vi "Example_LabVIEW_Google_Map.vi"() -> ()   [LabVIEW 2020]
panel:
  in  "Your Google Maps API Key":string
  in  "Zoom in":bool
  in  "Zoom Out":bool
  in  "Location List":i32(listbox)
  in  "Home":bool
  in  "Go":bool
  in  "WebBrowser":refnum<k7>(container)
  # "Google-Maps URL API for LabVIEW"
  # "Create by Wiseio"
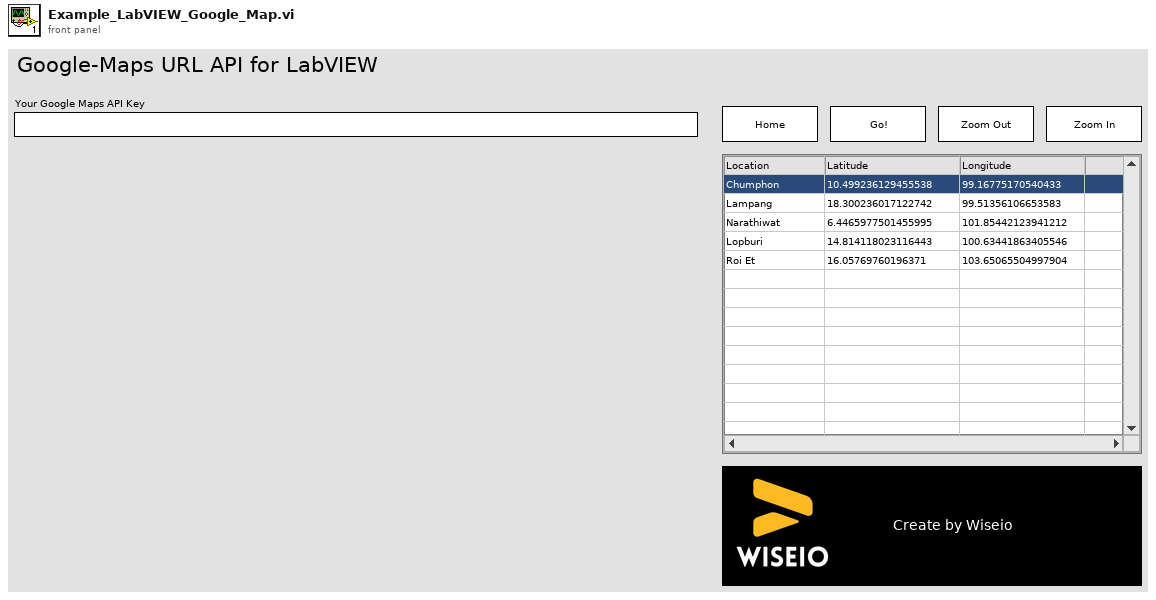
[diagram p1: front panel]
types:
  T1 = cluster{"Position":cluster{"Latitude":string, "Longitude":string}, "Color":string, "Character":string, "Size":string}
  T2 = cluster{"WebBrowser":refnum<k7>, "URL":string, "Parameter List":string[][]}
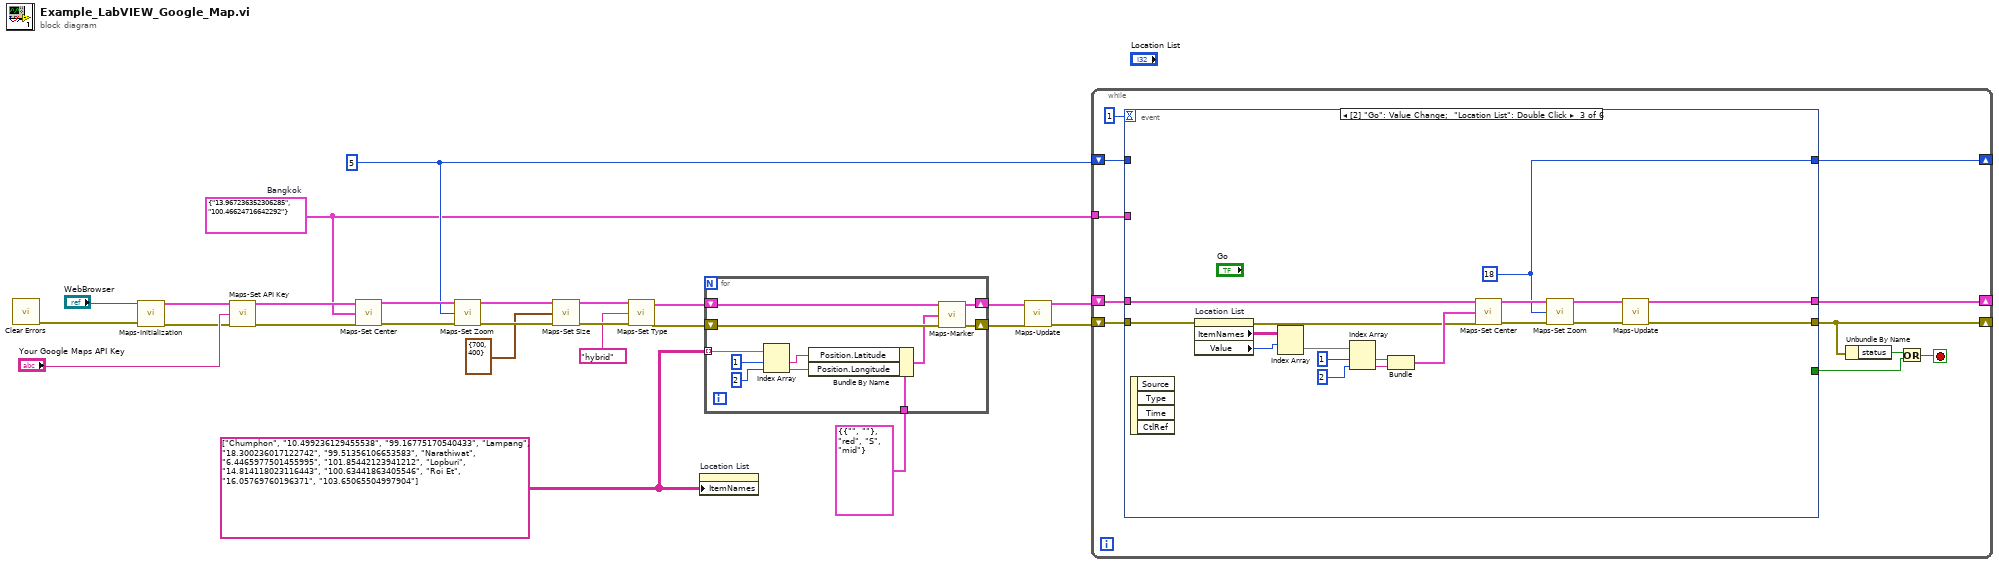
[diagram p0: block diagram]
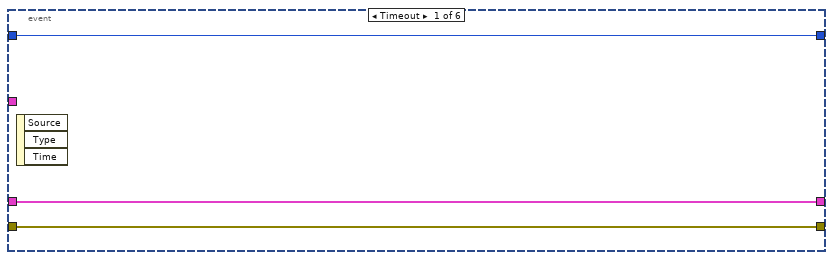
[diagram p2: hidden frame]
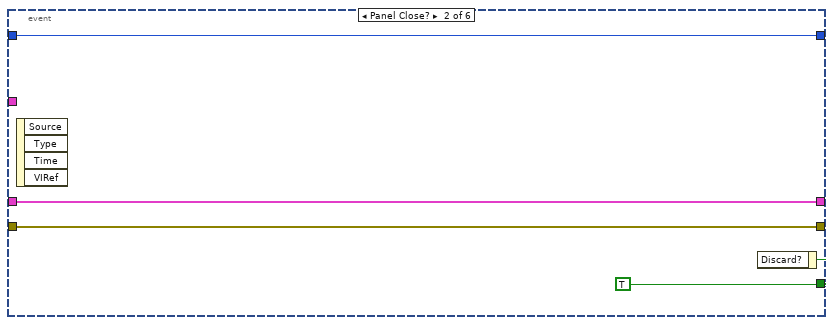
[diagram p3: hidden frame]
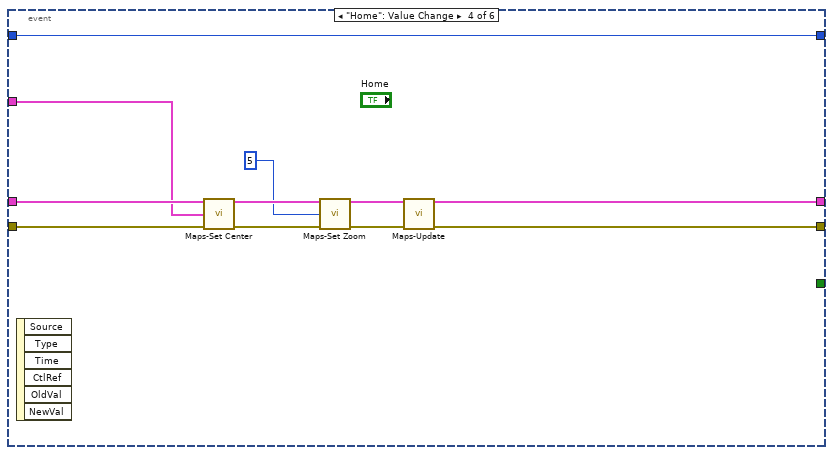
[diagram p4: hidden frame]
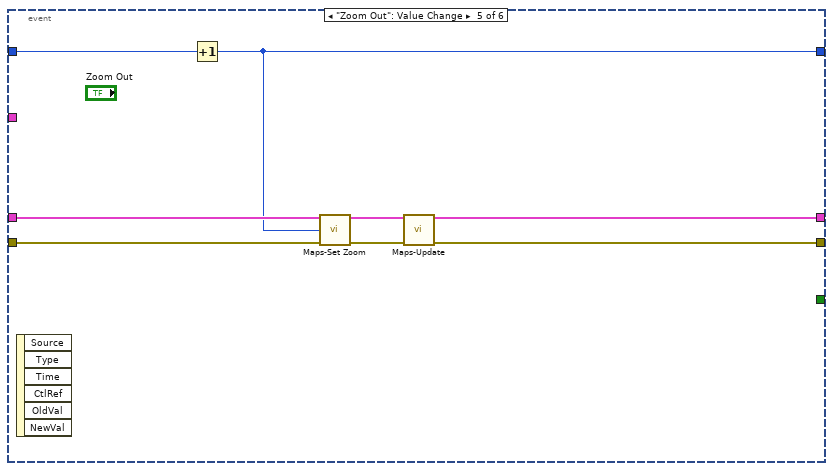
[diagram p5: hidden frame]
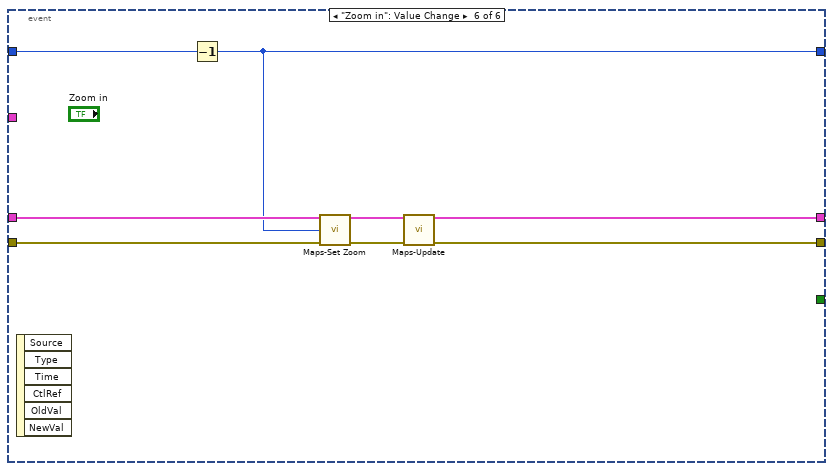
[diagram p6: hidden frame]
diagram:
  w1 = string[][] [["Chumphon", "10.499236129455538", "99.16775170540433"], ["Lampang", "18.300236017122742", "99.51356106653583"], ["Narathiwat", "6.4465977501455995", "101.85442123941212"], ["Lopburi", "14.814118023116443", "100.63441863405546"], ["Roi Et", "16.05769760196371", "103.65065504997904"]] ("Location List")
  w9 = 5 ("Zoom 2")
  w8 = cluster{"Latitude":string, "Longitude":string} {"Latitude"="13.967236352306285", "Longitude"="100.46624716642292"}  # Bangkok
  n1 = call <vilib>:"Clear Errors.vi"() -> ("error out"=w24:errorcluster)  [unwired: 6 in, 1 out]
  n2 = call "Maps-Initialization.vi"("Automation Refnum in"="WebBrowser", "error in (no error)"=w24) -> ("Google Maps Resource Out"=w22:T2, "error out"=w21:errorcluster)  [unwired: 12 in]
  n3 = call "Maps-Set API Key.vi"("Google Maps Resource Out in"=w22, "Google Maps API Key"="Your Google Maps API Key", "error in (no error)"=w21) -> ("Google Maps Resource Out out"=w11:T2, "error out"=w10:errorcluster)  [unwired: 11 in]
  n4 = call "Maps-Set Center.vi"("Google Maps Resource Out in"=w11, "Center Position"=w8, "error in (no error)"=w10) -> ("Google Maps Resource Out out"=w19:T2, "error out"=w18:errorcluster)  [unwired: 11 in]
  n5 = call "Maps-Set Zoom.vi"("Google Maps Resource Out in"=w19, "Zoom"=w9, "error in (no error)"=w18) -> ("Google Maps Resource Out out"=w17:T2, "error out"=w16:errorcluster)  [unwired: 11 in]
  n6 = call "Maps-Set Size.vi"("Google Maps Resource Out in"=w17, "Size"=cluster{"Width":i32, "Height":i32} {"Width"=700, "Height"=400} ("Size 2"), "error in (no error)"=w16) -> ("Google Maps Resource Out out"=w14:T2, "error out"=w13:errorcluster)  [unwired: 11 in]
  n7 = call "Maps-Set Type.vi"("Google Maps Resource Out in"=w14, "Type"="hybrid" ("Type 2"), "error in (no error)"=w13) -> ("Google Maps Resource Out out"=w7:T2, "error out"=w6:errorcluster)  [unwired: 11 in]
  n8 = property on="Location List" class="MCListbox (strict)"("ItemNames"=w1) -> ()  [unwired: 2 in, 2 out]
  n9 = for {
    shift-right: [w35] -> w5
    shift-left: w7 -> [w36]
    shift-right: [w33] -> w3
    shift-left: w6 -> [w34]
    tunnel: w1 -> [w32] mode=indexing
    tunnel: T1 {"Position"={"Latitude"="", "Longitude"=""}, "Color"="red", "Character"="S", "Size"="mid"} ("Marker") -> [w29]
    n10 = Index Array(array=w32, index #1=1 ("index"), index #2=2 ("index")) -> (element #1=w28:string, element #2=w27:string)
    n11 = Bundle By Name(cluster=w29, "Position.Latitude"=w28, "Position.Longitude"=w27) -> (w26:T1)
    n12 = call "Maps-Marker.vi"("Google Maps Resource Out in"=w36, "Marker"=w26, "error in (no error)"=w34) -> ("Google Maps Resource Out out"=w35:T2, "error out"=w33:errorcluster)  [unwired: 11 in]
  }
  n13 = call "Maps-Update.vi"("Google Maps Resource In"=w5, "error in (no error)"=w3) -> ("Google Maps Resource Out"=w4:T2, "error out"=w2:errorcluster)  [unwired: 11 in, 1 out]
  n14 = while {
    shift-right: [w44] -> _
    shift-left: w4 -> [w46]
    shift-right: [w43] -> _
    shift-left: w2 -> [w45]
    tunnel: w8 -> [w38]
    shift-right: [w37] -> _
    shift-left: w9 -> [w39]
    stop <- w41 stop-if-true
    n15 = event shown="[2] \"Go\": Value Change;  \"Location List\": Double Click" {
      selector: _ -> [_ _ _ _ _ _]
      dyn-events: _ -> [_ _ _ _ _ _]
      timeout: 1 -> [_ _ _ _ _ _]
      tunnel: w46 -> [w50 w54 w66 w82 w87 w95]
      tunnel: w45 -> [w49 w53 w72 w81 w86 w94]
      tunnel: [w50 w54 w56 w76 w89 w97] -> w44
      tunnel: [w49 w53 w57 w75 w88 w96] -> w43
      tunnel: [_ w52 _ _ _ _] -> w40
      tunnel: w39 -> [w48 w51 _ w74 w85 w93]
      tunnel: w38 -> [_ _ _ w80 _ _]
      tunnel: [w48 w51 w55 w74 w84 w92] -> w37
      event Timeout {
        n16 = event-data() -> ()  [unwired: 1 in, 3 out]
      }
      event Panel Close? {
        w52 = TRUE ("Discard?")
        n17 = event-data() -> ()  [unwired: 1 in, 4 out]
        n18 = event-data("Discard?"=w52) -> ()  [unwired: 1 in, 1 out]
      }
      event "Go": Value Change; "Location List": Double Click {
        w55 = 18 ("Zoom")
        n19 = event-data() -> ()  [unwired: 1 in, 4 out]
        n20 = property on="Location List" class="MCListbox (strict)"(error in=w72) -> (error out=w62:errorcluster, "ItemNames"=w71:string[][], "Value"=w70:i32)  [unwired: 1 in, 1 out]
        n21 = Index Array(array=w71, index (row)=w70) -> (element=w68:string[])  [unwired: 1 in]
        n22 = Index Array(array=w68, index #1=1 ("index"), index #2=2 ("index")) -> (element #1=w65:string, element #2=w64:string)
        n23 = Bundle(w65, w64) -> (w63:cluster{string, string})  [unwired: 1 in]
        n24 = call "Maps-Set Center.vi"("Google Maps Resource Out in"=w66, "Center Position"=w63, "error in (no error)"=w62) -> ("Google Maps Resource Out out"=w61:T2, "error out"=w60:errorcluster)  [unwired: 11 in]
        n25 = call "Maps-Set Zoom.vi"("Google Maps Resource Out in"=w61, "Zoom"=w55, "error in (no error)"=w60) -> ("Google Maps Resource Out out"=w59:T2, "error out"=w58:errorcluster)  [unwired: 11 in]
        n26 = call "Maps-Update.vi"("Google Maps Resource In"=w59, "error in (no error)"=w58) -> ("Google Maps Resource Out"=w56:T2, "error out"=w57:errorcluster)  [unwired: 11 in, 1 out]
      }
      event "Home": Value Change {
        n27 = event-data() -> ()  [unwired: 1 in, 6 out]
        n28 = call "Maps-Set Center.vi"("Google Maps Resource Out in"=w82, "Center Position"=w80, "error in (no error)"=w81) -> ("Google Maps Resource Out out"=w83:T2, "error out"=w79:errorcluster)  [unwired: 11 in]
        n29 = call "Maps-Set Zoom.vi"("Google Maps Resource Out in"=w83, "Zoom"=5 ("Zoom 2"), "error in (no error)"=w79) -> ("Google Maps Resource Out out"=w78:T2, "error out"=w77:errorcluster)  [unwired: 11 in]
        n30 = call "Maps-Update.vi"("Google Maps Resource In"=w78, "error in (no error)"=w77) -> ("Google Maps Resource Out"=w76:T2, "error out"=w75:errorcluster)  [unwired: 11 in, 1 out]
      }
      event "Zoom Out": Value Change {
        n31 = event-data() -> ()  [unwired: 1 in, 6 out]
        n32 = Increment(x=w85) -> (x+1=w84:i32)
        n33 = call "Maps-Set Zoom.vi"("Google Maps Resource Out in"=w87, "Zoom"=w84, "error in (no error)"=w86) -> ("Google Maps Resource Out out"=w91:T2, "error out"=w90:errorcluster)  [unwired: 11 in]
        n34 = call "Maps-Update.vi"("Google Maps Resource In"=w91, "error in (no error)"=w90) -> ("Google Maps Resource Out"=w89:T2, "error out"=w88:errorcluster)  [unwired: 11 in, 1 out]
      }
      event "Zoom in": Value Change {
        n35 = event-data() -> ()  [unwired: 1 in, 6 out]
        n36 = Decrement(x=w93) -> (x-1=w92:i32)
        n37 = call "Maps-Set Zoom.vi"("Google Maps Resource Out in"=w95, "Zoom"=w92, "error in (no error)"=w94) -> ("Google Maps Resource Out out"=w99:T2, "error out"=w98:errorcluster)  [unwired: 11 in]
        n38 = call "Maps-Update.vi"("Google Maps Resource In"=w99, "error in (no error)"=w98) -> ("Google Maps Resource Out"=w97:T2, "error out"=w96:errorcluster)  [unwired: 11 in, 1 out]
      }
    }
    n39 = Unbundle By Name(w43) -> ("status"=w42:bool)
    n40 = Or(x=w42, y=w40) -> (x .or. y?=w41:bool)
  }
